vi "verify.vi"(8 "error in (no error)":errorcluster, 11 "plugin_interface in":refnum<class "odbc_driver_postgres_v13.0.2.lvclass">) -> (0 "error out":errorcluster, 2 "installed?":bool, 3 "plugin_interface out":refnum<class "odbc_driver_postgres_v13.0.2.lvclass">)   [LabVIEW 2015, in "lv-example-postgres-post-installer.lvlib" / "odbc_driver_postgres_v13.0.2.lvclass"]
uses:
  odbc_driver_postgres_v13.0.2.lvclass
  <userlib>/antonio-alexander/lv-bin-windows/public/api/v1/v1.lvlib
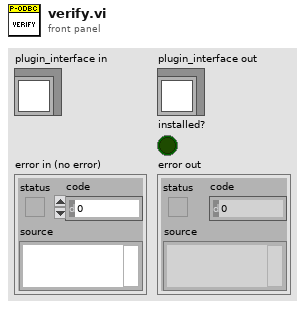
[diagram p1: front panel]
types:
  T1 = cluster{"display_name []":string[], "uninstall_string []":string[], "install_source []":string[], "install_location []":string[]}
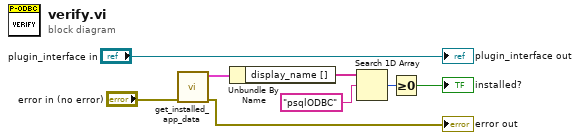
[diagram p0: block diagram]
diagram:
  n1 = call <userlib>:"get_installed_app_data.vi"("error in (no error)"="error in (no error)") -> ("error out"=→"error out":errorcluster, "installed_application_data []"=w4:T1)  [unwired: 9 in]
  n2 = Unbundle By Name(w4) -> ("display_name []"=w1:string[])
  n3 = Search 1D Array(1D array=w1, element="psqlODBC") -> (index of element=w2:i32)  [unwired: 1 in]
  n4 = Greater Or Equal To 0?(x=w2) -> (x >= 0?=→"installed?":bool)
  "plugin_interface out" <- "plugin_interface in"
